vi "WFS Calc Fourier Optometric.vi"(0 "instrument handle":refnum<visa-resource-name>, 5 "Zernike Orders":i32 format="%.0g", 7 "Fourier Order":i32 format="%.0g", 11 "error in (no error)":errorcluster {"code" format="%.0x"}) -> (3 "Opto Cylinder":dbl, 4 "instrument handle out":refnum<visa-resource-name>, 6 "Fourier M":dbl, 8 "Fourier J0":dbl, 10 "Fourier J45":dbl, 13 "Opto Axis deg":dbl, 14 "Opto Sphere":dbl, 15 "error out":errorcluster {"code" format="%.0x"})   [LabVIEW 2020]
doc: "This VI calculates the Fourier and Optometric notations from the Zernike coefficients calculated in WFS Zernike Lsf.vi.\n\nNote: WFS Zernike Lsf.vi is required to run prior to this VI."
uses:
  WFS_32.dll
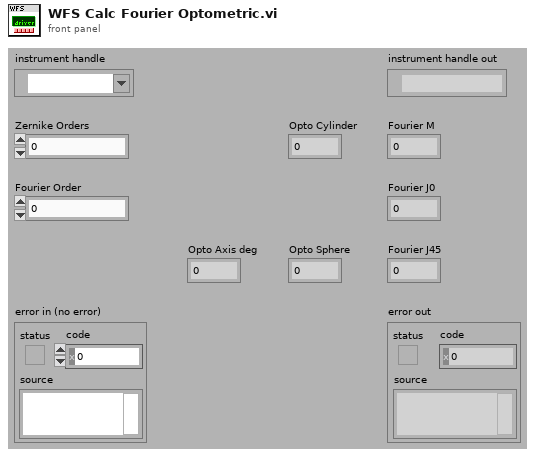
[diagram p1: front panel]
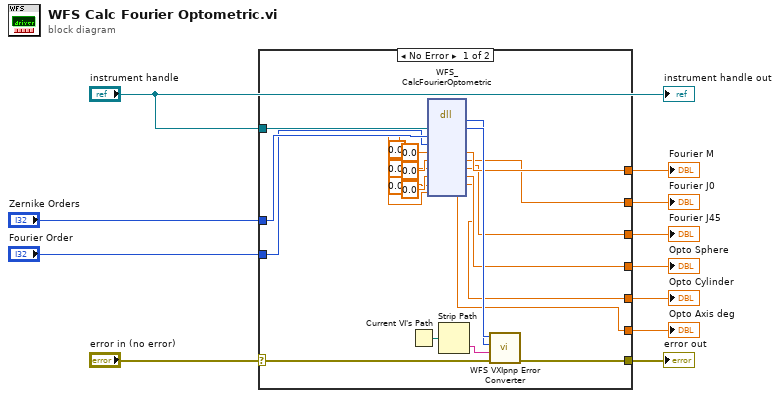
[diagram p0: block diagram]
diagram:
  n1 = case shown="No Error" "error in (no error)" {
    selector: "error in (no error)" -> [w27 w33]
    tunnel: [w26 w33] -> w11
    tunnel: "instrument handle" -> [w31 _]
    tunnel: "Zernike Orders" -> [w25 _]
    tunnel: "Fourier Order" -> [w24 _]
    tunnel: [w22 _] -> w6
    tunnel: [w20 _] -> w5
    tunnel: [w18 _] -> w4
    tunnel: [w16 _] -> w3
    tunnel: [w14 _] -> w2
    tunnel: [w12 _] -> w1
    frame No Error {
      n2 = Current VI's Path() -> (path=w32:path)
      n3 = dll-call lib="WFS_*.*" fn="WFS_CalcFourierOptometric"("Instrument Handle"=w31, "Zernike Orders"=w25, "Fourier Order"=w24, "Fourier M"=0.0, "Fourier J0"=0.0, "Fourier J45"=0.0, "Opto Sphere"=0.0, "Opto Cylinder"=0.0, "Opto Axis deg"=0.0) -> (w29:i32, "Instrument Handle"=w30:u32, "Fourier M"=w22:dbl, "Fourier J0"=w20:dbl, "Fourier J45"=w18:dbl, "Opto Sphere"=w16:dbl, "Opto Cylinder"=w14:dbl, "Opto Axis deg"=w12:dbl)  [unwired: 5 in, 2 out]
      n4 = Strip Path(path=w32) -> (name=w28:string)  [unwired: 1 out]
      n5 = call "WFS VXIpnp Error Converter.vi"("error in (no error)"=w27, "Name Of VI (\"\")"=w28, "CVI Error Code (0)"=w29, "instrument handle"=w30) -> ("error out"=w26:errorcluster)  [unwired: 6 in, 1 out]
    }
    frame Error {
    }
  }
  "error out" <- w11
  "Fourier M" <- w6
  "Fourier J0" <- w5
  "Fourier J45" <- w4
  "Opto Sphere" <- w3
  "Opto Cylinder" <- w2
  "Opto Axis deg" <- w1
  "instrument handle out" <- "instrument handle"
